vi "AndorSaveasSif.vi"(8 "error in":errorcluster, 10 "KinNumber":i32=10, 11 "FilePath":string="C:\\Users\\light\\Desktop\\Andor\\data") -> (0 "error out":errorcluster, 1 "FileName":string, 3 "SaveStatus":bool)   [LabVIEW 2014]
uses:
  <userlib>/atmcd64d.llb/Spool_method typedef.ctl
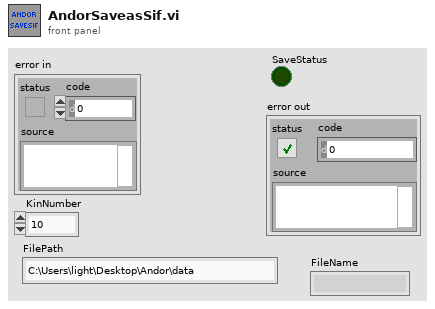
[diagram p1: front panel]
types:
  T1 = typedef "Spool_method typedef.ctl" = enum16{"32-bit", "Depends", "16-bit", "Multiple Directory", "Spool to RAM disk", "16-bit FITS", "SIF", "16-buit TIFF", "Multiple Directory Compressed"}
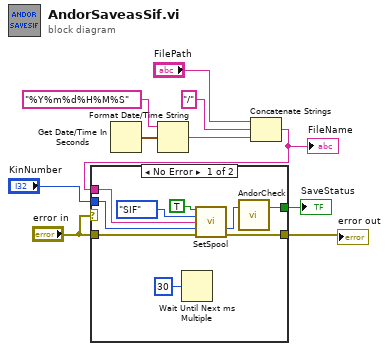
[diagram p0: block diagram]
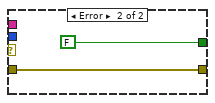
[diagram p2: hidden frame]
diagram:
  n1 = Get Date/Time In Seconds() -> (seconds since 1Jan1904=w4:timestamp)
  n2 = Format Date/Time String(time format string (%c)="%Y%m%d%H%M%S", seconds (now)=w4) -> (date/time string=w3:string)  [unwired: 1 in]
  n3 = Concatenate Strings("FilePath", "/" ("string"), w3) -> (w1:string)
  "FileName" <- w1
  n4 = case shown="No Error" "error in" {
    tunnel: "error in" -> [w17 w20]
    tunnel: [w15 FALSE ("Status")] -> w8
    tunnel: [w14 w20] -> w7
    tunnel: w1 -> [w13 _]
    tunnel: "KinNumber" -> [w12 _]
    frame No Error {
      n5 = Wait Until Next ms Multiple(millisecond multiple=u32 30) -> ()  [unwired: 1 out]
      n6 = call <userlib>:"SetSpool.vi"("active"=TRUE, "method"=Spool_method_typedef."SIF", "name"=w13, "framebuffersize (10)"=w12, "error in (no error)"=w17) -> ("DLL error code"=w16:u32, "error out"=w14:errorcluster)  [unwired: 9 in]
      n7 = call "AndorCheck.vi"("Input"=w16) -> ("Status"=w15:bool)  [unwired: 1 in, 1 out]
    }
    frame Error {
    }
  }
  "SaveStatus" <- w8
  "error out" <- w7
